vi "Set Configuration.vi"(8 "error in (no error)":errorcluster, 10 "plugin settings":T1, 11 "RDMA Plugin Configuration in":refnum<class "RDMA Plugin Configuration.lvclass">) -> (0 "error out":errorcluster, 3 "RDMA Plugin Configuration out":refnum<class "RDMA Plugin Configuration.lvclass">)   [LabVIEW 2020, in "RDMA.lvlib" / "RDMA Plugin Configuration.lvclass"]
uses:
  RDMA Plugin Configuration.lvclass
  Plugin Settings.ctl
  RDMA Plugin Configuration.lvclass/RDMA Plugin Configuration.ctl
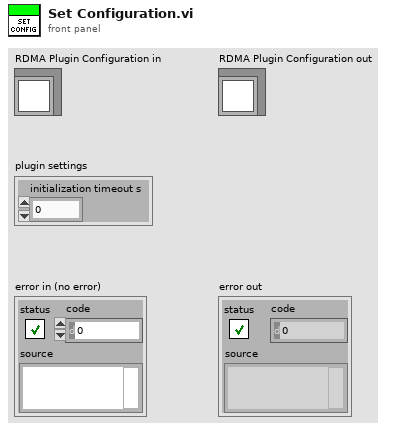
[diagram p1: front panel]
types:
  T1 = typedef "RDMA.lvlib/RDMA Plugin Configuration.lvclass/Plugin Settings.ctl" = cluster{"initialization timeout s":dbl}
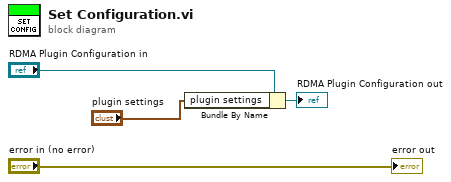
[diagram p0: block diagram]
diagram:
  n1 = Bundle By Name(cluster="RDMA Plugin Configuration in", "plugin settings"="plugin settings") -> (→"RDMA Plugin Configuration out":refnum<class "RDMA Plugin Configuration.lvclass">)
  "error out" <- "error in (no error)"
